vi "InfoH.vi"(11 "info":T1) -> ()   [LabVIEW 2014]
uses:
  Controls/infoHandle.ctl
  <vilib>/rvi/interface/RandomDataEmulation/niFpgaRandomDataHandleErrors.vi
  <vilib>/rvi/DataTransferAndStorage/Container/XNode/niFpgaContainer.xnode
  <vilib>/rvi/interface/RandomDataEmulation/nirviRandomDataFpgaReadWriteTemplate.vi
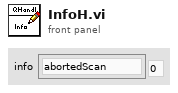
[diagram p1: front panel]
types:
  T1 = typedef "infoHandle.ctl" = enum16{"abortedScan", "stepComplete", "newScan", "newBunch"}
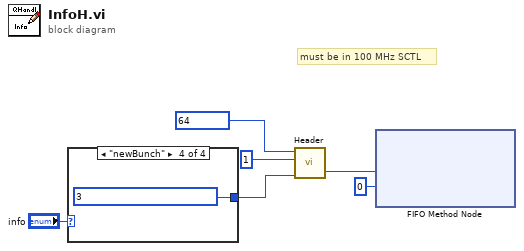
[diagram p0: block diagram]
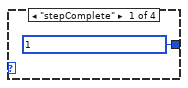
[diagram p2: hidden frame]
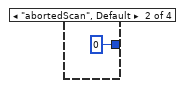
[diagram p3: hidden frame]
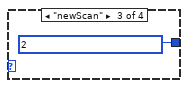
[diagram p4: hidden frame]
diagram:
  # "must be in 100 MHz SCTL"
  n1 = case shown="\"newBunch\"" "info" {
    tunnel: [u32 1 ("8BitHead") u32 0 ("8BitHead") u32 2 ("8BitHead") u32 3 ("8BitHead")] -> w2
    frame "stepComplete" {
    }
    frame "abortedScan", Default {
    }
    frame "newScan" {
    }
    frame "newBunch" {
    }
  }
  n2 = call "Header.vi"("23BitData"=w2, "1BitHeaderIndex"=u8 1, "8BitHead"=u8 64) -> ("32BitOutput"=w4:u32)  [unwired: 2 in]
  n3 = xnode ("FIFO Method Node")("Element"=w4, "Timeout"=0) -> ()  [unwired: 1 in, 2 out]
